vi "XPathTableStuff.vi"() -> ()   [LabVIEW 2013]
uses:
  XML.lvlib
  <vilib>/xml/NI_XML.lvlib
panel:
  in  "XPath":string="/text:p"
  out "XML":string[](array[string])=["<text:p xmlns:text=\"urn:oasis:names:tc:opendocument:xmlns:text:1.0\">Title1</text:p>"]
  out "error out":errorcluster
  in  "String":string="<table:table-row xmlns:table=\"urn:oasis:names:tc:opendocument:xmlns:table:1.0\" table:style-name=\"ro1\"><table:table-cell xmlns:calcext=\"urn:org:documentfoundation:names:experimental:calc:xmlns:calcext:1.0\" calcext:value-type=\"string\" xmlns:office=\"urn:oasis:names:tc:opendocument:xmlns:office:1.0\" office:value-type=\"string\"><text:p xmlns:text=\"urn:oasis:names:tc:opendocument:xmlns:text:1.0\">Title1</text:p></table:table-cell><table:table-cell table:number-columns-repeated=\"12\"/></table:table-row>"
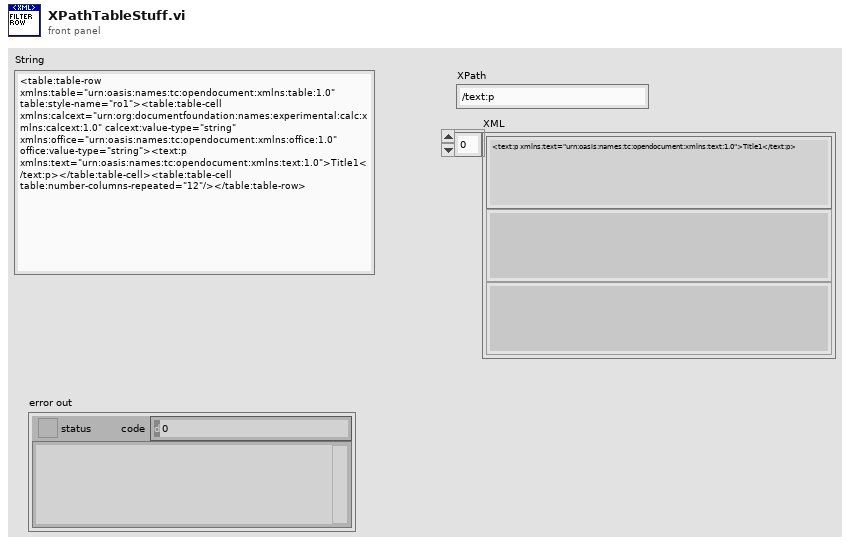
[diagram p1: front panel]
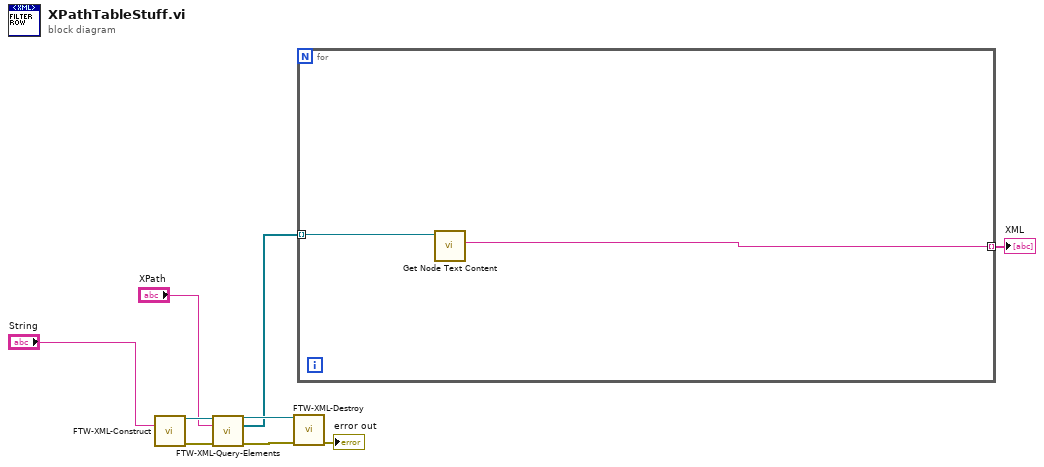
[diagram p0: block diagram]
diagram:
  n1 = call "FTW-XML-Construct.vi"("XML String"="String") -> ("XML Document"=w6:refnum<k20>, "error out"=w9:errorcluster)  [unwired: 13 in]
  n2 = call "FTW-XML-Query-Elements.vi"("XML Node"=w6, "XPath Query"="XPath", "error in"=w9) -> ("XML Node out"=w5:refnum<k20>, "Matching Nodes"=w3:refnum<k20>[], "error out"=w8:errorcluster)  [unwired: 9 in, 1 out]
  n3 = call "FTW-XML-Destroy.vi"("XML Node"=w5, "error in"=w8) -> ("error out"=→"error out":errorcluster)  [unwired: 13 in]
  n4 = for {
    tunnel: w3 -> [w11] mode=indexing
    tunnel: [w10] -> w1 mode=indexing
    n5 = call <vilib>:"Get Node Text Content.vi"("node in"=w11) -> ("node text"=w10:string)  [unwired: 8 in, 2 out]
  }
  "XML" <- w1
